vi "Detect Modules.vi"(8 "error in":errorcluster, 11 "Controller in":refnum<class "Controller.lvclass">) -> (0 "error out":errorcluster, 3 "Controller out":refnum<class "Controller.lvclass">)   [LabVIEW 2015]
uses:
  <vilib>/rvi/interface/nirviCloseFPGA/nirviCloseFPGA.xnode
  <vilib>/FPGAPlugInAG/Dynamic/niLvFpga_Close_Dynamic.vi
  Chassis/Chassis.lvclass
  Controller.lvclass
  <vilib>/regexp/Match Regular Expression.xnode
  Distributed Devices/Controls/DeviceInformation.ctl
panel:
  out "Modules":T1[](array[typedef]) {"Product ID" format="%.0x"}
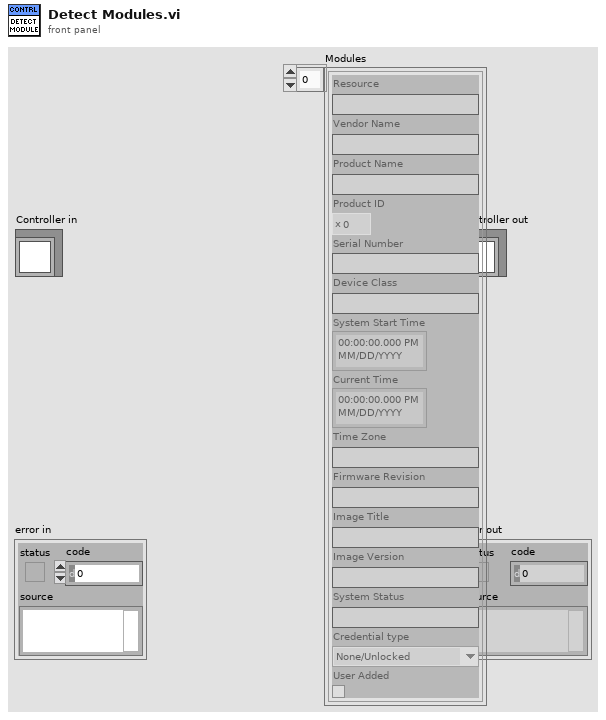
[diagram p1: front panel]
types:
  T1 = typedef "SMI.lvlib/Device.lvclass/DeviceInformation.ctl" = cluster{"Resource":string, "Vendor Name":string, "Product Name":string, "Product ID":u32, "Serial Number":string, "Device Class":string, "System Start Time":timestamp, "Current Time":timestamp, "Time Zone":string, "Firmware Revision":string, "Image Title":string, "Image Version":string, "System Status":string, "Credential type":enum16{"None/Unlocked", "FTP Password", "NIAuth Credentials"}, "User Added":bool}
  T2 = typedef "ModuleInformation.ctl" = cluster{"Vendor":string, "Model":string, "Module Code":u32, "Serial Number":string}
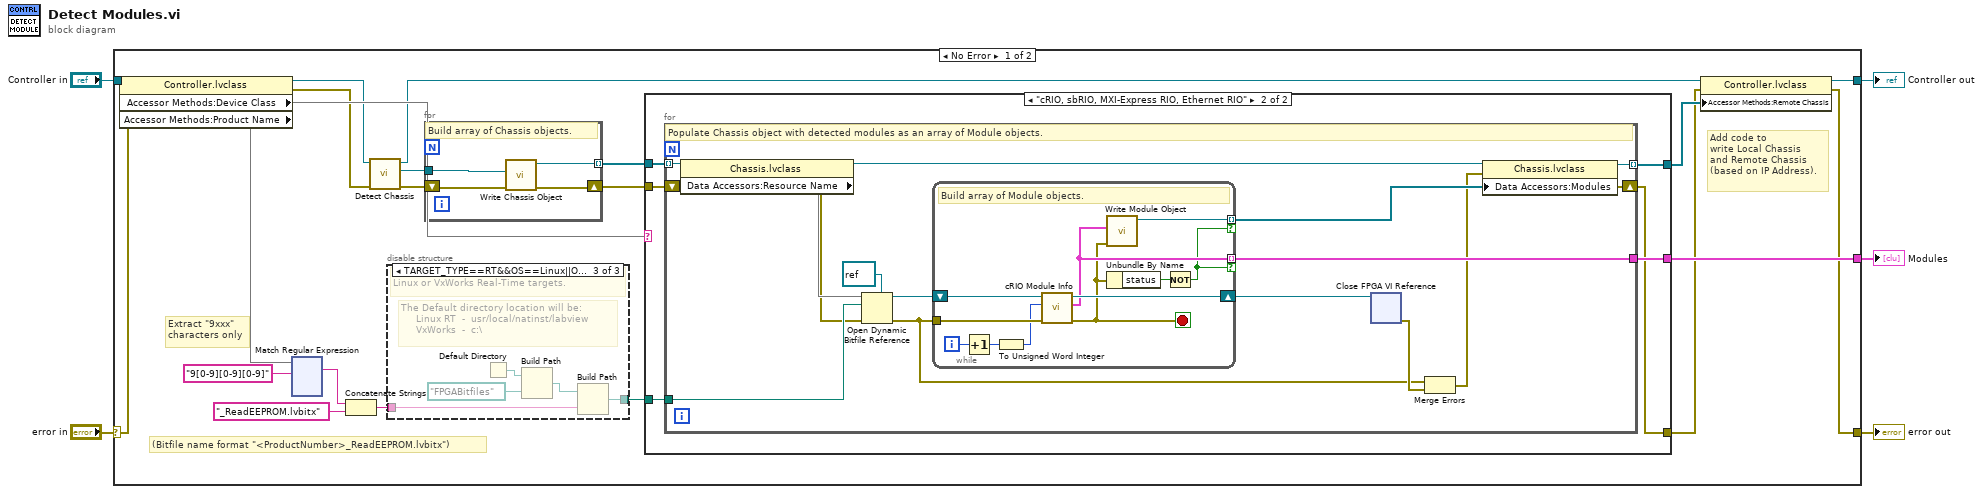
[diagram p0: block diagram]
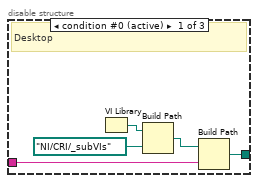
[diagram p2: hidden frame]
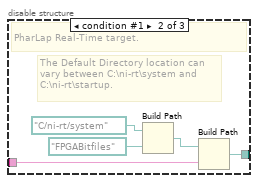
[diagram p3: hidden frame]
diagram:
  n1 = case shown="No Error" "error in" {
    selector: "error in" -> [w23 w195]
    tunnel: [w17 w195] -> w1
    tunnel: [w18 w194] -> w3
    tunnel: "Controller in" -> [w26 w194]
    tunnel: [w22 _] -> w2
    frame No Error {
      # "Extract \"9xxx\"\ncharacters only"
      # "Add code to\nwrite Local Chassis\nand Remote Chassis\n(based on IP Address)."
      # "(Bitfile name format \"<ProductNumber>_ReadEEPROM.lvbitx\")"
      n2 = property class="Controller.lvclass"(reference=w26, error in=w23) -> (reference out=w14:refnum<class "Controller.lvclass">, error out=w16:errorcluster, "Accessor Methods:Device Class"=w24, "Accessor Methods:Product Name"=w11)
      n3 = xnode "Match Regular Expression"("input string"=w11, "regular expression"="9[0-9][0-9][0-9]") -> ("whole match"=w10:string)  [unwired: 4 in, 4 out]
      n4 = Concatenate Strings(w10, "_ReadEEPROM.lvbitx" ("string")) -> (w6:string)
      n5 = call "Detect Chassis.vi"("error in"=w16, "Device in"=w14) -> ("error out"=w15:errorcluster, "Controller out"=w12:refnum<class "Controller.lvclass">, "Device out"=w13:refnum<class "Controller.lvclass">)  [unwired: 5 in, 2 out]
      n6 = disable-structure shown="TARGET_TYPE==RT&&OS==Linux||OS==VxWorks" {
        disable-tunnel: w6 -> [w31 w36 w41]
        disable-tunnel: [w30 w35 w40] -> w7
        frame condition #0 (active) {
          # "Desktop"
          n7 = VI Library() -> (path=w29:path)
          n8 = Build Path(base path=w29, name or relative path=path "NI/CRI/_subVIs") -> (appended path=w27:path)
          n9 = Build Path(base path=w27, name or relative path=w31) -> (appended path=w30:path)
        }
        frame condition #1 {
          # "The Default Directory location can\nvary between C:\\ni-rt\\system and\nC:\\ni-rt\\startup."
          # "PharLap Real-Time target."
          n10 = Build Path(base path=path "C:/ni-rt/system", name or relative path=path "FPGABitfiles") -> (appended path=w34:path)
          n11 = Build Path(base path=w34, name or relative path=w36) -> (appended path=w35:path)
        }
        frame condition #2 {
          # "The Default directory location will be:\n     Linux RT  -  usr/local/natinst/labview\n     VxWorks  -  c:\\"
          # "Linux or VxWorks Real-Time targets."
          n12 = Default Directory() -> (w37:path)
          n13 = Build Path(base path=w37, name or relative path=path "FPGABitfiles") -> (appended path=w39:path)
          n14 = Build Path(base path=w39, name or relative path=w41) -> (appended path=w40:path)
        }
      }
      n15 = for {
        tunnel: w12 -> [w158]
        tunnel: [w159] -> w21 mode=indexing
        shift-right: [w157] -> w8
        shift-left: w15 -> [w156]
        # "Build array of Chassis objects."
        n16 = call "Write Chassis Object.vi"("error in"=w156, "Chassis Information"=w158) -> ("error out"=w157:errorcluster, "Chassis out"=w159:refnum<class "Chassis.lvclass">)  [unwired: 8 in]
      }
      n17 = case shown="\"cRIO, sbRIO, MXI-Express RIO, Ethernet RIO\"" w24 {
        tunnel: w8 -> [w160 w166]
        tunnel: w7 -> [_ w165]
        tunnel: [w160 w163] -> w19
        tunnel: [_ w164] -> w22
        tunnel: w21 -> [_ w162]
        tunnel: [_ w161] -> w20
        frame Default {
        }
        frame "cRIO, sbRIO, MXI-Express RIO, Ethernet RIO" {
          n18 = for {
            tunnel: w165 -> [w182]
            tunnel: [w179] -> w164
            shift-right: [w172] -> w163
            shift-left: w166 -> [w169]
            tunnel: w162 -> [w177] mode=indexing
            tunnel: [w174] -> w161 mode=indexing
            # "Populate Chassis object with detected modules as an array of Module objects."
            n19 = property class="Chassis.lvclass"(reference=w177, error in=w169) -> (reference out=w176:refnum<class "Chassis.lvclass">, error out=w170:errorcluster, "Data Accessors:Resource Name"=w171)
            n20 = Open Dynamic Bitfile Reference(0:w171, 1:w182, 3:w170, 4:refnum<k20> refnum ("Refnum in")) -> (5:w167:refnum<k20>, 8:w168:errorcluster)  [unwired: 1 in]
            n21 = while {
              shift-right: [w192] -> w181
              shift-left: w167 -> [w189]
              tunnel: [w186] -> w179 mode=indexing if=w184
              tunnel: [w185] -> w175 mode=indexing if=w184
              tunnel: w168 -> [w193]
              i -> [w191]
              stop <- w183 stop-if-true
              # "Build array of Module objects."
              n22 = Increment(x=w191) -> (x+1=w187:i32)
              n23 = To Unsigned Word Integer(number=w187) -> (unsigned 16bit integer=w190:u16)
              n24 = call "cRIO Module Info.vi"("error in"=w193, "Slot (1-N)"=w190, "Refnum in"=w189) -> ("error out"=w183:errorcluster, "Module Information"=w186:T2, "Refnum out"=w192:refnum<k20>)  [unwired: 6 in]
              n25 = call "Write Module Object.vi"("error in"=w183, "Module Information"=w186) -> ("Module Detection out"=w185:refnum<class "Module Detection.lvclass">)  [unwired: 8 in, 1 out]
              n26 = Unbundle By Name(w183) -> ("status"=w188:bool)
              n27 = Not(x=w188) -> (.not. x?=w184:bool)
            }
            n28 = xnode "Close FPGA VI Reference"("FPGA VI Reference In"=w181) -> ("error out"=w178:errorcluster)  [unwired: 1 in]
            n29 = Merge Errors(w168, w178) -> (w173:errorcluster)
            n30 = property class="Chassis.lvclass"(reference=w176, error in=w173, "Data Accessors:Modules"=w175) -> (reference out=w174:refnum<class "Chassis.lvclass">, error out=w172:errorcluster)
          }
        }
      }
      n31 = property class="Controller.lvclass"(reference=w13, error in=w19, "Accessor Methods:Remote Chassis"=w20) -> (reference out=w18:refnum<class "Controller.lvclass">, error out=w17:errorcluster)
    }
    frame Error {
    }
  }
  "error out" <- w1
  "Controller out" <- w3
  "Modules" <- w2
